vi "TSM SSC Digital Configure Single Level Per-Site.vi"(0 "Digital TSM In":T2, 5 "Level Type to Set":T1, 7 "Per-Site Value":dbl[](array[numeric]), 11 "error in":errorcluster) -> (4 "Digital TSM Out":T2, 15 "error out":errorcluster)   [LabVIEW 2019]
doc: "Configures and applies the specified per-site levels to the specified pin(s) and pin group(s)."
uses:
  TSM/TSM SSC Digital.ctl
  <vilib>/NI_TestStand_SemiconductorModule/NI_TestStand_Semiconductor_Module.lvlibp/PinMap/Digital Pattern/PinQueryContext/DigitalPatternPinQueryContext.lvclass
  SSC Digital/SSC Digital.ctl
  SSC Digital/Pin Levels and Timing/SSC Digital Single Level Selection.ctl
  3e2341a4-810f-4dc2-85bd-7dde85c8f5db.vi
  Shared SubVIs/Site List to Site Numbers.vi
  Shared SubVIs/Channel List to Pins.vi
  Shared SubVIs/Trim Whitespace [Inlined].vi
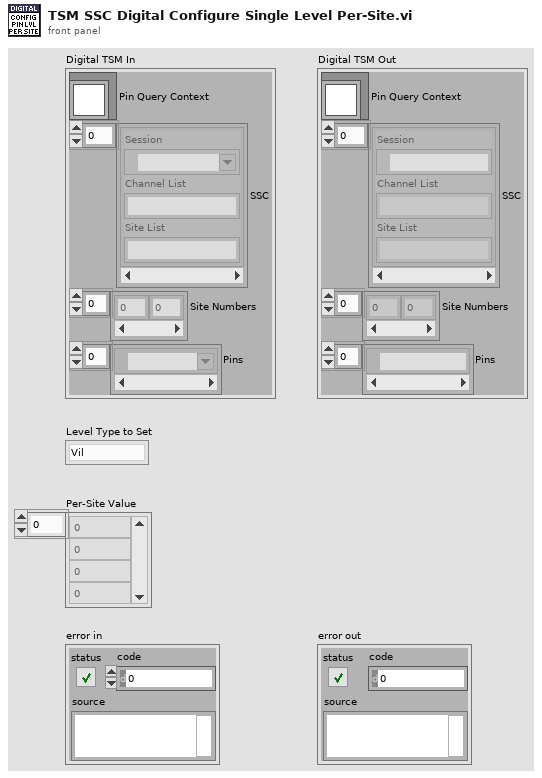
[diagram p1: front panel]
types:
  T1 = typedef "SSC Digital Single Level Selection.ctl" = enum16{"Vil", "Vih", "Vol", "Voh", "Vterm", "Iol", "Ioh", "Vcom"}
  T2 = typedef "TSM SSC Digital.ctl" = cluster{"Pin Query Context":refnum<class "DigitalPatternPinQueryContext.lvclass">, "SSC":T3[], "Site Numbers":i32[], "Pins":tag[]}
  T3 = typedef "SSC Digital.ctl" = cluster{"Session":refnum<k15>, "Channel List":string, "Site List":string}
  T4 = typedef "Digital 2D Location.ctl" = cluster{"Row":i32, "Col":i32}
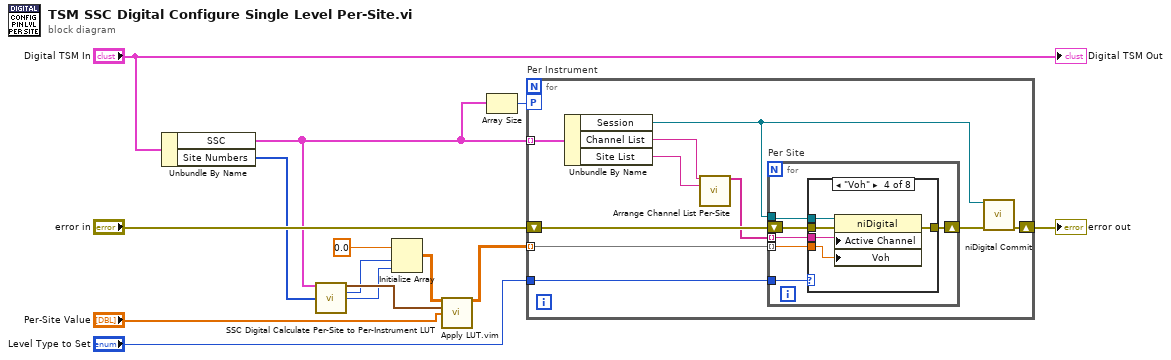
[diagram p0: block diagram]
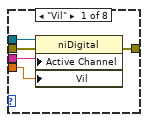
[diagram p2: hidden frame]
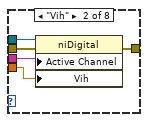
[diagram p3: hidden frame]
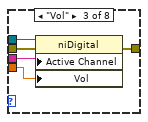
[diagram p4: hidden frame]
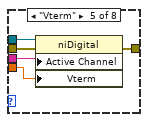
[diagram p5: hidden frame]
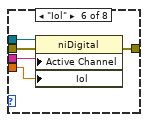
[diagram p6: hidden frame]
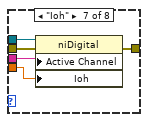
[diagram p7: hidden frame]
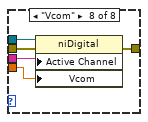
[diagram p8: hidden frame]
diagram:
  n1 = Unbundle By Name("Digital TSM In") -> ("SSC"=w1:T3[], "Site Numbers"=w5:i32[])
  n2 = call "SSC Digital Calculate Per-Site to Per-Instrument LUT.vi"("Digital SSC In"=w1, "Sites"=w5) -> ("Per-Site to Per-Instrument LUT"=w9:T4[], "Instrument Count"=w8:i32, "Max Sites on Instrument"=w7:i32)  [unwired: 11 in]
  n3 = Initialize Array(0.0 ("element"), w8, w7) -> (w11:dbl[][])
  n4 = call "Apply LUT.vim"("Initialized Array"=w11, "LUT"=w9, "Results to Apply LUT to"="Per-Site Value") -> ("Array Out"=w3:dbl[][])  [unwired: 12 in]
  n5 = Array Size(array=w1) -> (size(s)=w2:i32)
  n6 = for "Per Instrument" {
    workers-P: w2 -> [_]
    tunnel: w3 -> [w15] mode=indexing
    tunnel: "Level Type to Set" -> [w21]
    tunnel: w1 -> [w20] mode=indexing
    shift-right: [w22] -> w14
    shift-left: "error in" -> [w24]
    n7 = Unbundle By Name(w20) -> ("Session"=w19:refnum<k15>, "Channel List"=w18:string, "Site List"=w17:string)
    n8 = call "Arrange Channel List Per-Site.vi"("Channel List String"=w18, "Site List String"=w17) -> ("Channel List Array"=w16:string[])  [unwired: 11 in, 2 out]
    n9 = for "Per Site" {
      tunnel: w21 -> [w28]
      tunnel: w19 -> [w27]
      tunnel: w16 -> [w26] mode=indexing
      shift-right: [w29] -> w23
      shift-left: w24 -> [w30]
      tunnel: w15 -> [w25] mode=indexing
      n10 = case shown="\"Voh\"" w28 {
        tunnel: w30 -> [w35 w40 w45 w50 w55 w60 w65 w70]
        tunnel: [w34 w39 w44 w49 w54 w59 w64 w69] -> w29
        tunnel: w27 -> [w33 w38 w43 w48 w53 w58 w63 w68]
        tunnel: w26 -> [w32 w37 w42 w47 w52 w57 w62 w67]
        tunnel: w25 -> [w31 w36 w41 w46 w51 w56 w61 w66]
        frame "Vil" {
          n11 = property on="Property Node" class="niDigital"(reference=w33, error in=w35, "Active Channel"=w32, "Vil"=w31) -> (error out=w34:errorcluster)  [unwired: 1 out]
        }
        frame "Vih" {
          n12 = property on="Property Node" class="niDigital"(reference=w38, error in=w40, "Active Channel"=w37, "Vih"=w36) -> (error out=w39:errorcluster)  [unwired: 1 out]
        }
        frame "Vol" {
          n13 = property on="Property Node" class="niDigital"(reference=w43, error in=w45, "Active Channel"=w42, "Vol"=w41) -> (error out=w44:errorcluster)  [unwired: 1 out]
        }
        frame "Voh" {
          n14 = property on="Property Node" class="niDigital"(reference=w48, error in=w50, "Active Channel"=w47, "Voh"=w46) -> (error out=w49:errorcluster)  [unwired: 1 out]
        }
        frame "Vterm" {
          n15 = property on="Property Node" class="niDigital"(reference=w53, error in=w55, "Active Channel"=w52, "Vterm"=w51) -> (error out=w54:errorcluster)  [unwired: 1 out]
        }
        frame "Iol" {
          n16 = property on="Property Node" class="niDigital"(reference=w58, error in=w60, "Active Channel"=w57, "Iol"=w56) -> (error out=w59:errorcluster)  [unwired: 1 out]
        }
        frame "Ioh" {
          n17 = property on="Property Node" class="niDigital"(reference=w63, error in=w65, "Active Channel"=w62, "Ioh"=w61) -> (error out=w64:errorcluster)  [unwired: 1 out]
        }
        frame "Vcom" {
          n18 = property on="Property Node" class="niDigital"(reference=w68, error in=w70, "Active Channel"=w67, "Vcom"=w66) -> (error out=w69:errorcluster)  [unwired: 1 out]
        }
      }
    }
    n19 = call <instrlib>:"niDigital Commit.vi"("instrument handle"=w19, "error in"=w23) -> ("error out"=w22:errorcluster)  [unwired: 12 in, 1 out]
  }
  "error out" <- w14
  "Digital TSM Out" <- "Digital TSM In"
